vi "MP3音乐播放器实验.vi"() -> ()   [LabVIEW 2011]
uses:
  <vilib>/STM32_DriverVI_Interface_F4/FATFS/File Style_F4.ctl
  <vilib>/STM32_DriverVI_Interface_F4/MP3/MP3 Sound Effect_F4.ctl
  <vilib>/STM32_DriverVI_Interface_F4/MP3/MP3 Forward Backward_F4.ctl
panel:
  in  "快退":bool
  in  "快进":bool
  out "进度（%）":dbl
  out "Play Prograss（S）":u16
  out "Total Time (S)":dbl
  in  "暂停":bool
  out "Open_Success?":bool
  out "file_path":string="0:PICTURE"
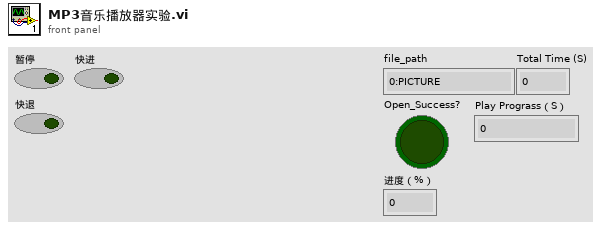
[diagram p1: front panel]
types:
  T1 = enum8{"P0", "P1", "P2", "P3", "P4", "P5", "P6", "P7", "P8", "P9", "P10", "P11", "P12", "P13", "P14", "P15"}
  T2 = enum8{"Port_A", "Port_B", "Port_C", "Port_D", "Port_E", "Port_F", "Port_G", "Port_H", "Port_I"}
  T3 = typedef "File Style_F4.ctl" = u8
  T4 = typedef "MP3 Sound Effect_F4.ctl" = enum8{"关闭", "最小", "中等", "最大"}
  T5 = typedef "MP3 Forward Backward_F4.ctl" = enum8{"Forward Fast", "Backward Fast"}
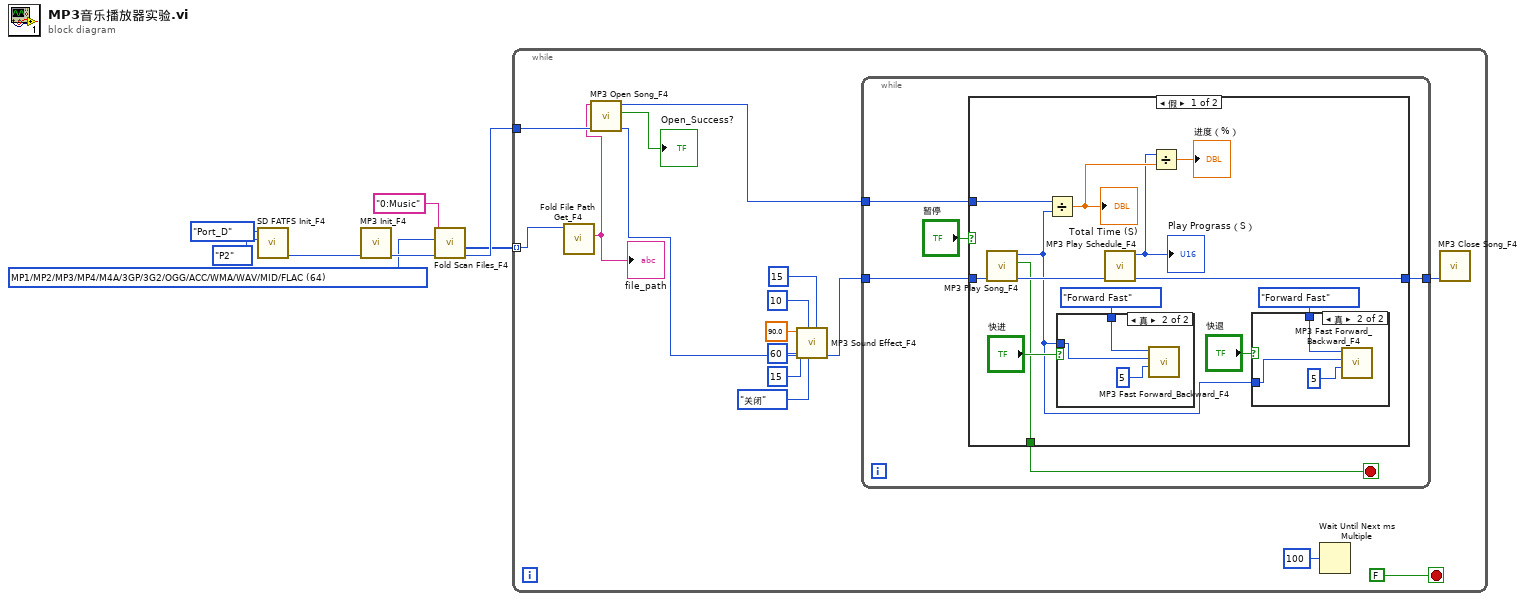
[diagram p0: block diagram]
diagram:
  w5 = T3 64 items=[".BIN"=0, ".LRC"=16, ".NES"=32, ".TXT/.C/.H"=48, "MP1/MP2/MP3/MP4/M4A/3GP/3G2/OGG/ACC/WMA/WAV/MID/FLAC"=64, ".BMP/.JPG/.JPEG/.GIF"=80] ("File Type")
  n1 = call <vilib>:"SD FATFS Init_F4.vi"("SD_CS_pin"=T1."P2", "SD_CS_PortX"=T2."Port_D") -> ("err_out"=w3:u8)  [unwired: 8 in, 1 out]
  n2 = call <vilib>:"MP3 Init_F4.vi"("err_in"=w3) -> ("err_out"=w8:u8)  [unwired: 10 in]
  n3 = call <vilib>:"Fold Scan Files_F4.vi"("err_in"=w8, "File Type"=w5, "fold_path"="0:Music") -> ("err_out"=w7:u8, "files_index"=w4:u16[])  [unwired: 5 in, 2 out]
  n4 = while {
    tunnel: w7 -> [w22]
    tunnel: w4 -> [w21] mode=indexing
    stop <- FALSE stop-if-true
    n5 = call <vilib>:"Fold File Path Get_F4.vi"("File Index"=w21) -> ("file_path"=w20:string)  [unwired: 8 in, 2 out]
    "file_path" <- w20
    n6 = call <vilib>:"MP3 Open Song_F4.vi"("err_in"=w22, "Music File Path"=w20) -> ("err_out"=w17:u8, "Open_Success?"=→"Open_Success?":bool, "Music Total Size（Kb）"=w19:u32)  [unwired: 7 in]
    n7 = call <vilib>:"MP3 Sound Effect_F4.vi"("高频增益（1.5 dB）"=u8 15, "MP3 Sound Effect"=MP3_Sound_Effect_F4."关闭", "高频下限频率（KHz）"=u8 10, "err_in"=w17, "低频增益（1 dB）"=u8 15, "低频上限频率（Hz）"=u8 60, "Volume（%）"=90.0) -> ("err_out"=w10:u8)  [unwired: 4 in]
    n8 = while {
      tunnel: w19 -> [w28]
      tunnel: w10 -> [w27]
      tunnel: [w26] -> w9
      stop <- w25 stop-if-true
      n9 = case shown="假" "暂停" {
        tunnel: w28 -> [w41 _]
        tunnel: w27 -> [w42 _]
        tunnel: [w37 _] -> w26
        tunnel: [w30 _] -> w25
        frame False {
          n10 = call <vilib>:"MP3 Play Song_F4.vi"("err_in"=w42) -> ("err_out"=w40:u8, "Play Over？"=w30:bool, "Decoder_Speed（Kbps）"=w31:u16)  [unwired: 8 in]
          n11 = Divide(x=w41, y=w31) -> (x/y=w39:dbl)
          "Total Time (S)" <- w39
          n12 = case shown="真" "快进" {
            tunnel: MP3_Forward_Backward_F4."Forward Fast" ("MP3 Forward/Backward") -> [_ w48]
            tunnel: w31 -> [_ w47]
            frame False {
            }
            frame True {
              n13 = call <vilib>:"MP3 Fast Forward_Backward_F4.vi"("Step Time（s）"=u16 5, "Decoder_Speed（Kbps）"=w47, "MP3 Forward/Backward"=w48) -> ()  [unwired: 8 in, 1 out]
            }
          }
          n14 = call <vilib>:"MP3 Play Schedule_F4.vi"("err_in"=w40) -> ("err_out"=w37:u8, "Play Prograss（S）"=w38:u16)  [unwired: 9 in]
          "Play Prograss（S）" <- w38
          n15 = Divide(x=w38, y=w39) -> (x/y=→"进度（%）":dbl)
          n16 = case shown="真" "快退" {
            tunnel: MP3_Forward_Backward_F4."Forward Fast" ("MP3 Forward/Backward") -> [_ w45]
            tunnel: w31 -> [_ w44]
            frame False {
            }
            frame True {
              n17 = call <vilib>:"MP3 Fast Forward_Backward_F4.vi"("Step Time（s）"=u16 5, "Decoder_Speed（Kbps）"=w44, "MP3 Forward/Backward"=w45) -> ()  [unwired: 8 in, 1 out]
            }
          }
        }
        frame True {
        }
      }
    }
    n18 = Wait Until Next ms Multiple(millisecond multiple=u32 100 ("毫秒倍数")) -> ()  [unwired: 1 out]
    n19 = call <vilib>:"MP3 Close Song_F4.vi"("err_in"=w9) -> ()  [unwired: 9 in, 2 out]
  }
